vi "P541_Ctrl_Index.vi"(5 "OldVal":variant, 11 "NewVal":variant) -> (4 "Control out":refnum<vi>, 8 "P541 Out":T1)   [LabVIEW 2014]
uses:
  Type Defs/P541.ctl
panel:
  in  "P541 In":T1
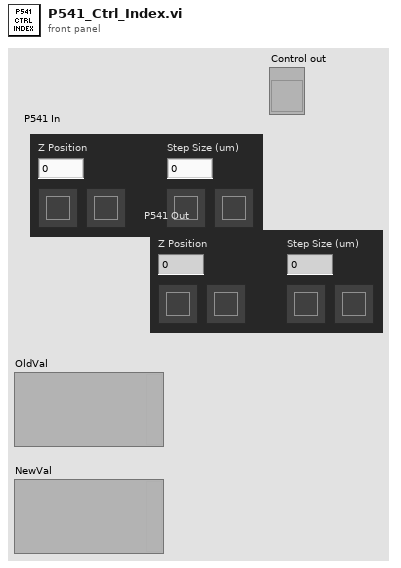
[diagram p1: front panel]
types:
  T1 = typedef "P541.ctl" = cluster{"Step Up":bool, "Step Down":bool, "Z Position":dbl, "Step Size (um)":dbl, "Home":bool, "Save":bool}
  T2 = cluster{"Step Up":bool, "Step Down":bool, "Z Position":bool, "Step Size (um)":bool, "Home":bool, "Save":bool}
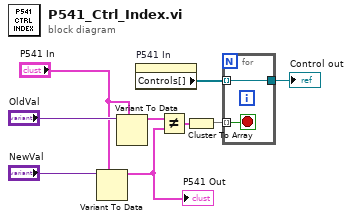
[diagram p0: block diagram]
diagram:
  n1 = Variant To Data(type="P541 In", Variant="NewVal") -> (data=w9:T1)  [unwired: 1 in, 1 out]
  "P541 Out" <- w9
  n2 = Variant To Data(type="P541 In", Variant="OldVal") -> (data=w4:T1)  [unwired: 1 in, 1 out]
  n3 = property on="P541 In" class="Clust"() -> ("Controls[]"=w1:refnum<vi>[])  [unwired: 2 in, 2 out]
  n4 = Not Equal?(x=w4, y=w9) -> (x != y?=w8:T2)
  n5 = Cluster To Array(cluster=w8) -> (array=w5:bool[])
  n6 = for {
    tunnel: w5 -> [w10] mode=indexing
    tunnel: w1 -> [w11] mode=indexing
    tunnel: [w11] -> w3
    stop <- w10 stop-if-true
  }
  "Control out" <- w3
